vi "CSMP-Template.vi"(0 "state":string, 1 "args":string, 2 "source/target":string, 3 "Pre-State":string, 4 "Pre-Args":string, 5 "Error in":errorcluster caption="Error in (no error)", 7 "Response Timeout(5000ms)":i32, 8 "Module Name":string) -> (14 "state out":string, 15 "args out":string, 16 "source/target out":string, 17 "Pre-State out":string, 18 "Pre-Args out":string, 19 "error":errorcluster)   [LabVIEW 2014, in "Communicable State Machine.lvlib"]
uses:
  Priority Queue/Priority Queue.lvclass/Priority Queue.ctl
  Typedef/_Cross CSM State Data.ctl
  Typedef/_CSM_MSG_TYPE.ctl
  Typedef/_Cross CSM State Response.ctl
  Typedef/_CSM_Response Source Message.ctl
  Common/CSM-Name to CSM-Mode.vi
  Priority Queue/Not a Refnum.vi
  CSMQ/_CSMOFGV.vi
  Communicable State Machine.lvlib
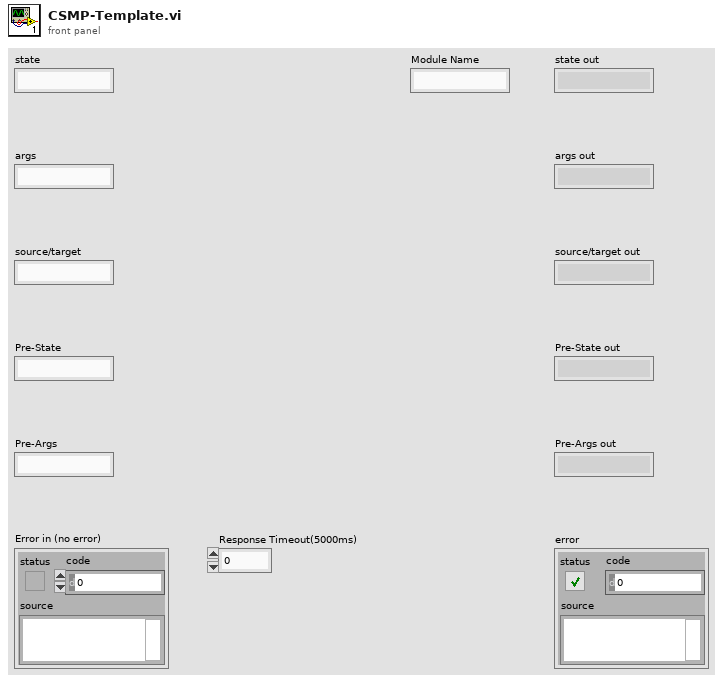
[diagram p1: front panel]
types:
  T1 = typedef "Communicable State Machine.lvlib/_CSMObj.ctl" = cluster{"Queue Name":string, "Mode":T2, "Share Count":i32, "Queue":refnum<class "Priority Queue.lvclass">, "Locked Status":refnum<data-value>, "User Event":refnum<user-event>, "Status Change Event":refnum<user-event>}
  T2 = typedef "Communicable State Machine.lvlib/_CSM_MODE.ctl" = enum16{"Stand Alone", "CSM", "Action Worker"}
  T3 = typedef "Communicable State Machine.lvlib/_Cross CSM State Response.ctl" = cluster{"error":errorcluster, "Response Data":string, "From Who":string}
  T4 = typedef "Communicable State Machine.lvlib/_CSM_MSG_TYPE.ctl" = enum16{"Sync Message(-@)", "Async Message(->)", "Async without Response(->|)", "Async Response", "Broadcast(-><status>)", "Broadcast(-><interrupt>)", "Request to Post Message", "Request to Post Message without Reply", "Request to Publish Status"}
  T5 = typedef "Communicable State Machine.lvlib/_Cross CSM State Data.ctl" = cluster{"Msg Type":T4, "state":string, "args":string, "source":string, "RespQ":refnum<queue>, "Response For Message":T6, "Target":string}
  T6 = typedef "Communicable State Machine.lvlib/_CSM_Response Source Message.ctl" = cluster{"State":string, "Arguments":string, "Error":errorcluster}
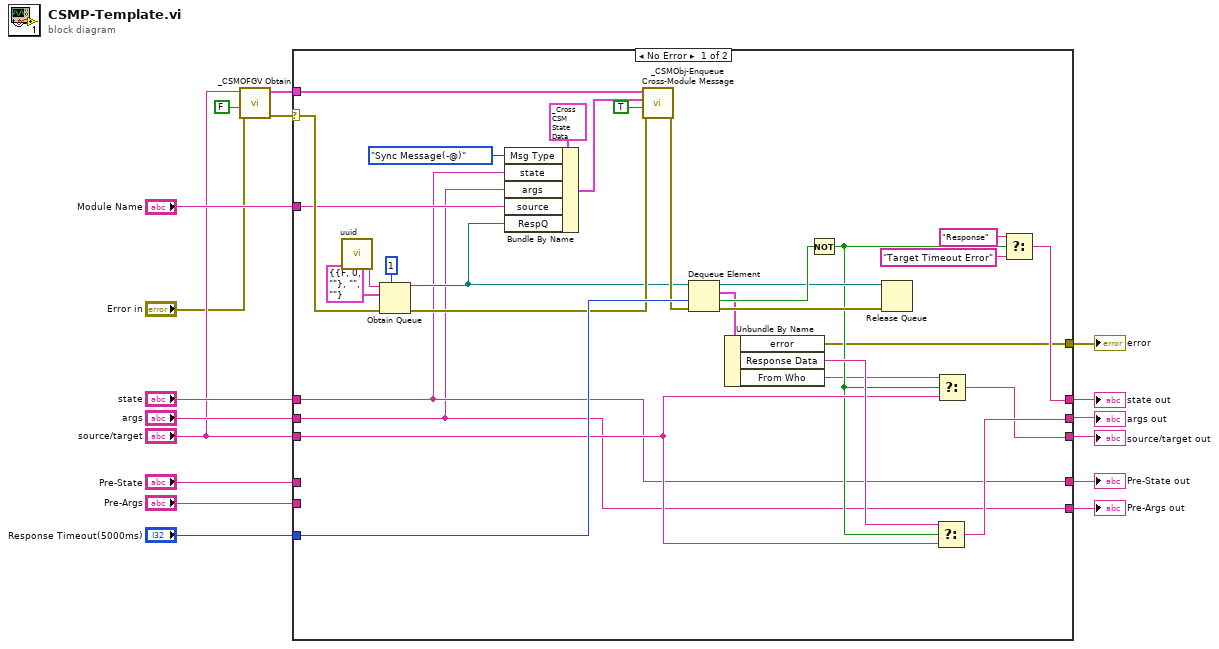
[diagram p0: block diagram]
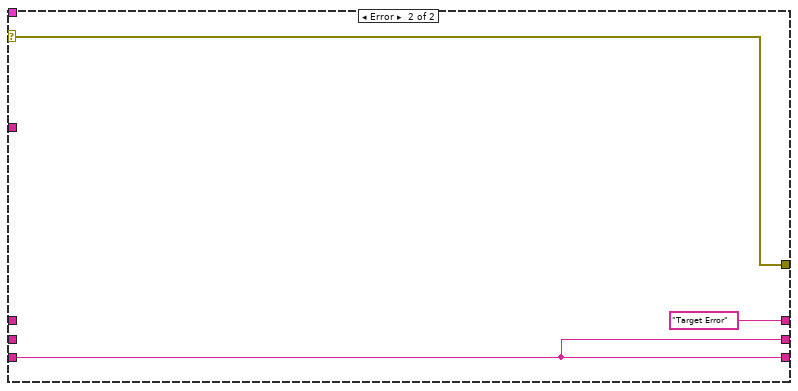
[diagram p2: hidden frame]
diagram:
  n1 = call "_CSMOFGV Obtain.vi"("Error in"="Error in", "create if not found? (T)"=FALSE, "Name(\"\" to use uuid) in"="source/target") -> ("Error out"=w16:errorcluster, "CSM-Obj"=w17:T1)  [unwired: 5 in, 2 out]
  n2 = case shown="No Error" w16 {
    selector: w16 -> [w38 w48]
    tunnel: "Response Timeout(5000ms)" -> [w46 _]
    tunnel: w17 -> [w47 _]
    tunnel: [w45 "Target Error" ("before match")] -> w9
    tunnel: [w31 w49] -> w8
    tunnel: "source/target" -> [w27 w49]
    tunnel: "state" -> [w20 _]
    tunnel: "args" -> [w18 _]
    tunnel: "Module Name" -> [w28 _]
    tunnel: [w18 _] -> w6
    tunnel: [w21 w48] -> w5
    tunnel: [w20 _] -> w7
    tunnel: "Pre-State" -> [_ _]
    tunnel: "Pre-Args" -> [_ _]
    tunnel: [w19 w49] -> w1
    frame No Error {
      n3 = call "uuid.vi"() -> ("UUID"=w22:string)  [unwired: 11 in]
      n4 = Obtain Queue(max queue size (-1, unlimited)=1, name (unnamed)=w22, element data type=T3 {"error"={"status"=FALSE, "code"=0, "source"=""}, "Response Data"="", "From Who"=""} ("Cross JKI State Machine Response"), error in (no error)=w38) -> (queue out=w30:refnum<queue>, error out=w34:errorcluster)  [unwired: 1 in, 1 out]
      n5 = Bundle By Name(cluster=T5 {"Msg Type"=enum."Sync Message(-@)", "state"="", "args"="", "source"="", "RespQ"=refnum, "Response For Message"={"State"="", "Arguments"="", "Error"={"status"=FALSE, "code"=0, "source"=""}}, "Target"=""} ("Cross JKI State Machine State"), "Msg Type"=_CSM_MSG_TYPE."Sync Message(-@)", "state"=w20, "args"=w18, "source"=w28, "RespQ"=w30) -> (w39:T5)
      n6 = call "_CSMObj-Enqueue Cross-Module Message.vi"("Error in"=w34, "High Priority?(F)"=TRUE, "Data"=w39, "CSMQ in"=w47) -> ("Error out"=w35:errorcluster)  [unwired: 5 in, 2 out]
      n7 = Dequeue Element(queue=w30, timeout in ms (-1)=w46, error in (no error)=w35) -> (queue out=w37:refnum<queue>, element=w33:T3, timed out?=w44:bool, error out=w36:errorcluster)
      n8 = Unbundle By Name(w33) -> ("error"=w21:errorcluster, "Response Data"=w32:string, "From Who"=w25:string)
      n9 = Not(x=w44) -> (.not. x?=w26:bool)
      n10 = Release Queue(queue=w37, error in (no error)=w36) -> ()  [unwired: 1 in, 3 out]
      n11 = Select(t=w32, s=w26, f=w27) -> (s? t:f=w31:string)
      n12 = Select(t=w25, s=w26, f=w27) -> (s? t:f=w19:string)
      n13 = Select(t="Response" ("f"), s=w26, f="Target Timeout Error" ("before match")) -> (s? t:f=w45:string)
    }
    frame Error {
    }
  }
  "state out" <- w9
  "args out" <- w8
  "source/target out" <- w1
  "Pre-State out" <- w7
  "Pre-Args out" <- w6
  "error" <- w5
